vi "Base.vi"(11 "Boolean input":bool) -> (3 "Boolean indicator":bool)   [LabVIEW 2025]
panel:
  in  "String inside a cluster":string
  in  "Cluster with a string inside it 2":cluster{"String inside a cluster":string}={"String inside a cluster"="12345"}
  in  "Cluster with a string inside it":cluster{}
  out "Text  indicator":string
  in  "A text indicator":string
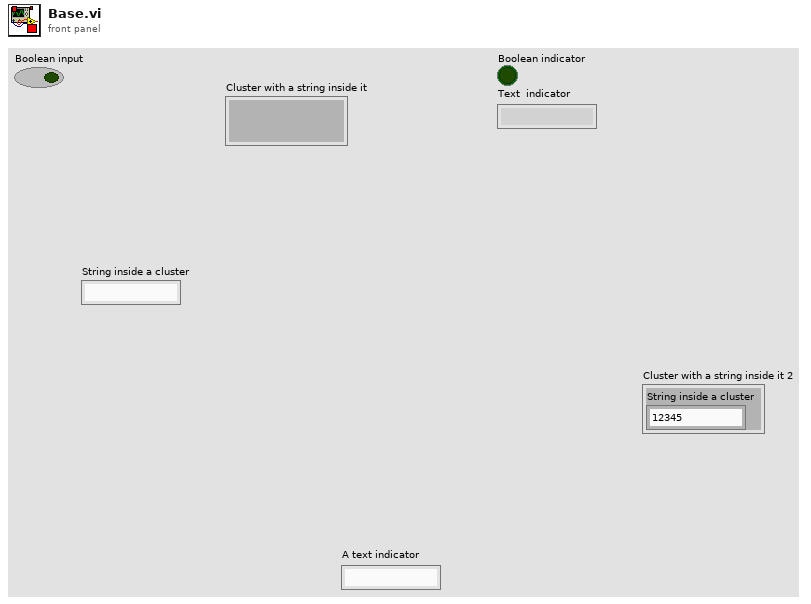
[diagram p1: front panel]
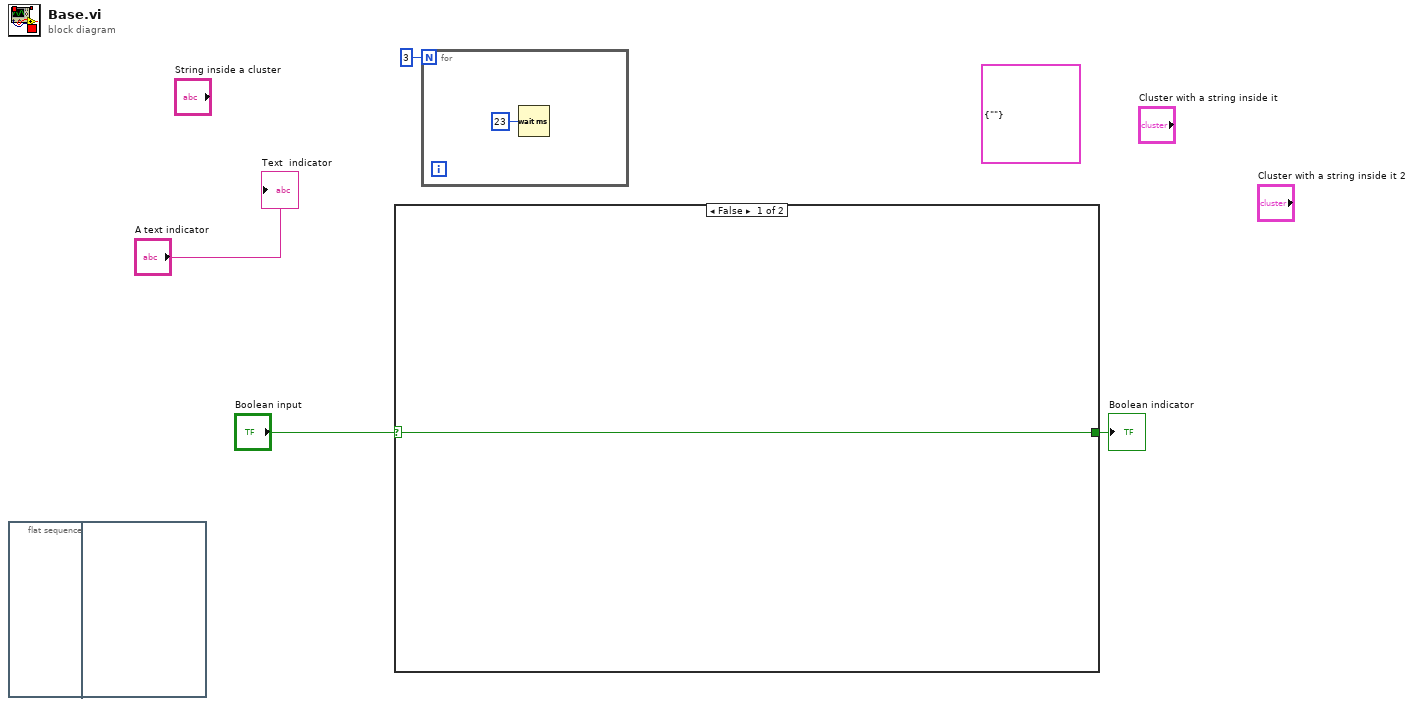
[diagram p0: block diagram]
diagram:
  (unwired) cluster{string} {""}
  n1 = flat-sequence {
    frame #0 {
    }
    frame #1 {
    }
  }
  n2 = case shown="False" "Boolean input" {
    selector: "Boolean input" -> [w5 w6]
    tunnel: [w5 w6] -> w3
    frame False {
    }
    frame True {
    }
  }
  "Boolean indicator" <- w3
  n3 = for {
    N: 3 -> [_]
    n4 = Wait (ms)(milliseconds to wait=u32 23) -> ()  [unwired: 1 out]
  }
  "Text  indicator" <- "A text indicator"
